vi "GetStatus.vi"(8 "error in (no error)":errorcluster, 11 "S4GUI in":refnum<class "S4GUI.lvclass">) -> (0 "error out":errorcluster, 3 "S4GUI out":refnum<class "S4GUI.lvclass">)   [LabVIEW 2018, in "S4GUI.lvclass"]
uses:
  S4GUI.lvclass
  S4GUI.lvclass/S4GUI.ctl
  Server/Server.lvclass/Server.ctl
  Instrument/Instrument.lvclass/Instrument.ctl
  Device/Optics/Optics.lvclass/Optics.ctl
  Interface/Interface.lvclass/Interface.ctl
  TelFocus/TelFocus.lvclass
  WeatherStation/WeatherStation.lvclass
  Instrument/Instrument.lvclass
  TCS/TCS.lvclass
  SyncBox/Sync Box.lvclass
  Device/Optics/Opt_Selector/Opt_Selector.lvclass
  Device/Optics/Opt_Continuous/Opt_Continuous.lvclass
  Acquisition/Acquisition.lvclass
  GSserver/GSserver.lvclass
  Channel/Channel.lvclass
  Interface/Interface.lvclass
  GSstatus/GSstatus.lvclass
  SecMirror/SecMirror.lvclass
  WeatherSensor/WeatherSensor.lvclass
  Trigger/Trigger.lvclass
  Device/Optics/Optics.lvclass
  Server/Server.lvclass
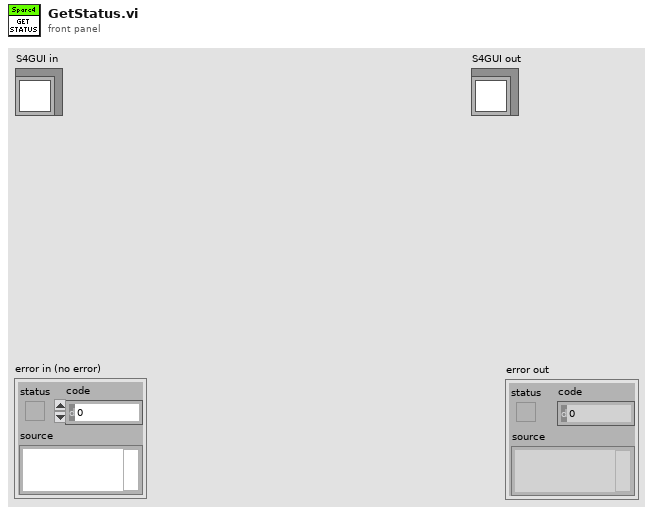
[diagram p1: front panel]
types:
  T1 = cluster{"ACQUISITION_MODE":bool, "TRIGGER_MODE":bool, "READ_MODE":bool, "PREAMP":bool, "READOUT_RATE":bool, "VERTICAL_SHIFT_SPEED":bool, "EM_MODE":bool, "EM_GAIN":bool, "SHUTTER_MODE":bool, "SHUTTER_TTL":bool, "SHUTTER_OPENING_TIME":bool, "SHUTTER_CLOSING_TIME":bool, "VBIN":bool, "HBIN":bool, "INITIAL_LINE":bool, "INITIAL_COLUMN":bool, "FINAL_LINE":bool, "FINAL_COLUMN":bool, "FRAME_TRANSFER":bool, "VERTICAL_CLOCK_VOLTAGE":bool, "AD_CHANNEL":bool}
  T2 = cluster{"ACQUISITION_MODE":u8, "TRIGGER_MODE":u8, "READ_MODE":u8, "PREAMP":u8, "READOUT_RATE":u8, "VERTICAL_SHIFT_SPEED":u8, "EM_MODE":u8, "EM_GAIN":u16, "SHUTTER_MODE":u8, "SHUTTER_TTL":u8, "SHUTTER_OPENING_TIME":u16, "SHUTTER_CLOSING_TIME":u16, "VBIN":u16, "HBIN":u16, "INITIAL_LINE":u16, "INITIAL_COLUMN":u16, "FINAL_LINE":u16, "FINAL_COLUMN":u16, "FRAME_TRANSFER":bool, "VERTICAL_CLOCK_VOLTAGE":u8, "AD_CHANNEL":u32}
  T3 = cluster{"Trigger Mode Status":string, "String output":string, "Instrument Status":cluster{"WPROT pos":dbl, "WPSEL pos":dbl, "GMIR pos":dbl, "GFOC pos":dbl, "CALW pos":dbl, "ASEL pos":dbl, "mode":bool, "String Status":string, "connection":bool, "operational":bool}, "Sync Box State":i32, "Trigger General Status":string, "Instrument States":cluster{"WPSEL State":i32, "WPROT State":i32, "CALW State":i32, "ASEL State":i32, "GMIR State":i32, "GFOC State":i32}, "Instrument Pos Names":cluster{"WPROT posname":string, "WPSEL posname":string, "CALW posname":string, "ASEL posname":string}, "ChannelA_Status":cluster{"Current exp":dbl, "Frames done":u32, "LastFileImage":string, "CamStatus":string, "Run state":u32, "connection":bool, "Cooler ON/OFF":i16, "Currently temperature":i16, "Temperature Status":string, "target  temp":i16, "conf runing":bool, "FT":bool, "UsedDisk":u16, "operational":bool}, "WPROT seq":u16, "ChannelB_Status":cluster{"Current exp":dbl, "Frames done":u32, "LastFileImage":string, "CamStatus":string, "Run state":u32, "connection":bool, "Cooler ON/OFF":i16, "Currently temperature":i16, "Temperature Status":string, "target  temp":i16, "conf runing":bool, "FT":bool, "UsedDisk":u16, "operational":bool}, "ChannelC_Status":cluster{"Current exp":dbl, "Frames done":u32, "LastFileImage":string, "CamStatus":string, "Run state":u32, "connection":bool, "Cooler ON/OFF":i16, "Currently temperature":i16, "Temperature Status":string, "target  temp":i16, "conf runing":bool, "FT":bool, "UsedDisk":u16, "operational":bool}, "ChannelD_Status":cluster{"Current exp":dbl, "Frames done":u32, "LastFileImage":string, "CamStatus":string, "Run state":u32, "connection":bool, "Cooler ON/OFF":i16, "Currently temperature":i16, "Temperature Status":string, "target  temp":i16, "conf runing":bool, "FT":bool, "UsedDisk":u16, "operational":bool}, "ChannelA_CCD":cluster{"ACQUISITION_MODE":u8, "TRIGGER_MODE":u8, "READ_MODE":u8, "PREAMP":u8, "READOUT_RATE":u8, "VERTICAL_SHIFT_SPEED":u8, "EM_MODE":u8, "EM_GAIN":u16, "SHUTTER_MODE":u8, "SHUTTER_TTL":u8, "SHUTTER_OPENNING_TIME":u16, "SHUTTER_CLOSING_TIME":u16, "VBIN":u16, "HBIN":u16, "INITIAL_LINE":u16, "INITIAL_COLUMN":u16, "FINAL_LINE":u16, "FINAL_COLUMN":u16, "FRAME_TRANSFER":bool, "VERTICAL_CLOCK_VOLTAGE":u8, "AD_CHANNEL":u32}, "ChannelB_CCD ":cluster{"ACQUISITION_MODE":u8, "TRIGGER_MODE":u8, "READ_MODE":u8, "PREAMP":u8, "READOUT_RATE":u8, "VERTICAL_SHIFT_SPEED":u8, "EM_MODE":u8, "EM_GAIN":u16, "SHUTTER_MODE":u8, "SHUTTER_TTL":u8, "SHUTTER_OPENNING_TIME":u16, "SHUTTER_CLOSING_TIME":u16, "VBIN":u16, "HBIN":u16, "INITIAL_LINE":u16, "INITIAL_COLUMN":u16, "FINAL_LINE":u16, "FINAL_COLUMN":u16, "FRAME_TRANSFER":bool, "VERTICAL_CLOCK_VOLTAGE":u8, "AD_CHANNEL":u32}, "ChannelC_CCD":cluster{"ACQUISITION_MODE":u8, "TRIGGER_MODE":u8, "READ_MODE":u8, "PREAMP":u8, "READOUT_RATE":u8, "VERTICAL_SHIFT_SPEED":u8, "EM_MODE":u8, "EM_GAIN":u16, "SHUTTER_MODE":u8, "SHUTTER_TTL":u8, "SHUTTER_OPENNING_TIME":u16, "SHUTTER_CLOSING_TIME":u16, "VBIN":u16, "HBIN":u16, "INITIAL_LINE":u16, "INITIAL_COLUMN":u16, "FINAL_LINE":u16, "FINAL_COLUMN":u16, "FRAME_TRANSFER":bool, "VERTICAL_CLOCK_VOLTAGE":u8, "AD_CHANNEL":u32}, "ChannelD_CCD":cluster{"ACQUISITION_MODE":u8, "TRIGGER_MODE":u8, "READ_MODE":u8, "PREAMP":u8, "READOUT_RATE":u8, "VERTICAL_SHIFT_SPEED":u8, "EM_MODE":u8, "EM_GAIN":u16, "SHUTTER_MODE":u8, "SHUTTER_TTL":u8, "SHUTTER_OPENNING_TIME":u16, "SHUTTER_CLOSING_TIME":u16, "VBIN":u16, "HBIN":u16, "INITIAL_LINE":u16, "INITIAL_COLUMN":u16, "FINAL_LINE":u16, "FINAL_COLUMN":u16, "FRAME_TRANSFER":bool, "VERTICAL_CLOCK_VOLTAGE":u8, "AD_CHANNEL":u32}, "CHA_Checked Params":cluster{"ACQUISITION_MODE":bool, "TRIGGER_MODE":bool, "READ_MODE":bool, "PREAMP":bool, "READOUT_RATE":bool, "VERTICAL_SHIFT_SPEED":bool, "EM_MODE":bool, "EM_GAIN":bool, "SHUTTER_MODE":bool, "SHUTTER_TTL":bool, "SHUTTER_OPENING_TIME":bool, "SHUTTER_CLOSING_TIME":bool, "VBIN":bool, "HBIN":bool, "INITIAL_LINE":bool, "INITIAL_COLUMN":bool, "FINAL_LINE":bool, "FINAL_COLUMN":bool, "FRAME_TRANSFER":bool, "VERTICAL_CLOCK_VOLTAGE":bool, "AD_CHANNEL":bool}, "CHB_Checked Params":cluster{"ACQUISITION_MODE":bool, "TRIGGER_MODE":bool, "READ_MODE":bool, "PREAMP":bool, "READOUT_RATE":bool, "VERTICAL_SHIFT_SPEED":bool, "EM_MODE":bool, "EM_GAIN":bool, "SHUTTER_MODE":bool, "SHUTTER_TTL":bool, "SHUTTER_OPENING_TIME":bool, "SHUTTER_CLOSING_TIME":bool, "VBIN":bool, "HBIN":bool, "INITIAL_LINE":bool, "INITIAL_COLUMN":bool, "FINAL_LINE":bool, "FINAL_COLUMN":bool, "FRAME_TRANSFER":bool, "VERTICAL_CLOCK_VOLTAGE":bool, "AD_CHANNEL":bool}, "CHC_Checked Params":cluster{"ACQUISITION_MODE":bool, "TRIGGER_MODE":bool, "READ_MODE":bool, "PREAMP":bool, "READOUT_RATE":bool, "VERTICAL_SHIFT_SPEED":bool, "EM_MODE":bool, "EM_GAIN":bool, "SHUTTER_MODE":bool, "SHUTTER_TTL":bool, "SHUTTER_OPENING_TIME":bool, "SHUTTER_CLOSING_TIME":bool, "VBIN":bool, "HBIN":bool, "INITIAL_LINE":bool, "INITIAL_COLUMN":bool, "FINAL_LINE":bool, "FINAL_COLUMN":bool, "FRAME_TRANSFER":bool, "VERTICAL_CLOCK_VOLTAGE":bool, "AD_CHANNEL":bool}, "CHD_Checked Params":cluster{"ACQUISITION_MODE":bool, "TRIGGER_MODE":bool, "READ_MODE":bool, "PREAMP":bool, "READOUT_RATE":bool, "VERTICAL_SHIFT_SPEED":bool, "EM_MODE":bool, "EM_GAIN":bool, "SHUTTER_MODE":bool, "SHUTTER_TTL":bool, "SHUTTER_OPENING_TIME":bool, "SHUTTER_CLOSING_TIME":bool, "VBIN":bool, "HBIN":bool, "INITIAL_LINE":bool, "INITIAL_COLUMN":bool, "FINAL_LINE":bool, "FINAL_COLUMN":bool, "FRAME_TRANSFER":bool, "VERTICAL_CLOCK_VOLTAGE":bool, "AD_CHANNEL":bool}, "Trigger_connection":bool, "TCSPD_connection":bool, "TCS extended":string, "TCS id":u32, "S4ICS id":u32, "focus pos":i32, "Focus_connection":bool, "WS_connection":bool, "weather status":cluster{"broker":string, "version":string, "date":string, "hour":string, "outHumidity":string, "inHumidity":string, "inTemp":string, "outTemp":string, "windSpeed":string, "windDirection":string, "pressure":string, "dewOut":string, "dewIn":string, "leaf":string, "rain":string, "windChill":string}, "GS STATUS cluster":cluster{"FocusPhot":dbl, "FocusPolar":dbl, "FocusEffic":dbl, "FocusInstrum":dbl, "ICS":bool, "AG":bool, "BROKER":string}, "TCSPD_operational":bool, "Focus_operational":bool, "object_suffix":string, "dflat_suffix":string, "sflat_suffix":string, "dark_suffix":string, "zero_suffix":string, "focus_suffix":string, "suffixAlertVisible":bool}
  T4 = cluster{"TEMP":dbl, "EXPTIME":dbl, "#FRAMES":u32, "#CYCLES":u32, "#SEQS":u32, "WAVEPLATE_POS":u32, "COOLER_POWER_STATUS":dbl, "suffix":string}
  T5 = cluster{"FocusPhot":dbl, "FocusPolar":dbl, "FocusEffic":dbl, "FocusInstrum":dbl, "ICS":bool, "AG":bool, "BROKER":string}
  T6 = cluster{"broker":string, "version":string, "date":string, "hour":string, "outHumidity":string, "intHumidity":string, "inTemp":string, "outTemp":string, "windSpeed":string, "windDirection":string, "pressure":string, "dewOut":string, "dewIn":string, "leaf":string, "rain":string, "windChill":string}
  T7 = cluster{"Texp":dbl, "Nimages":u32, "InitialLine":u32, "FinalLine":u32, "InitialColumn":u32, "FinalColumn":u32, "EmGain":u32, "Cooler Off":bool, "CyclesDone":u32, "SequesDone":u32, "UsedDiskSpace":u16, "Error":bool}
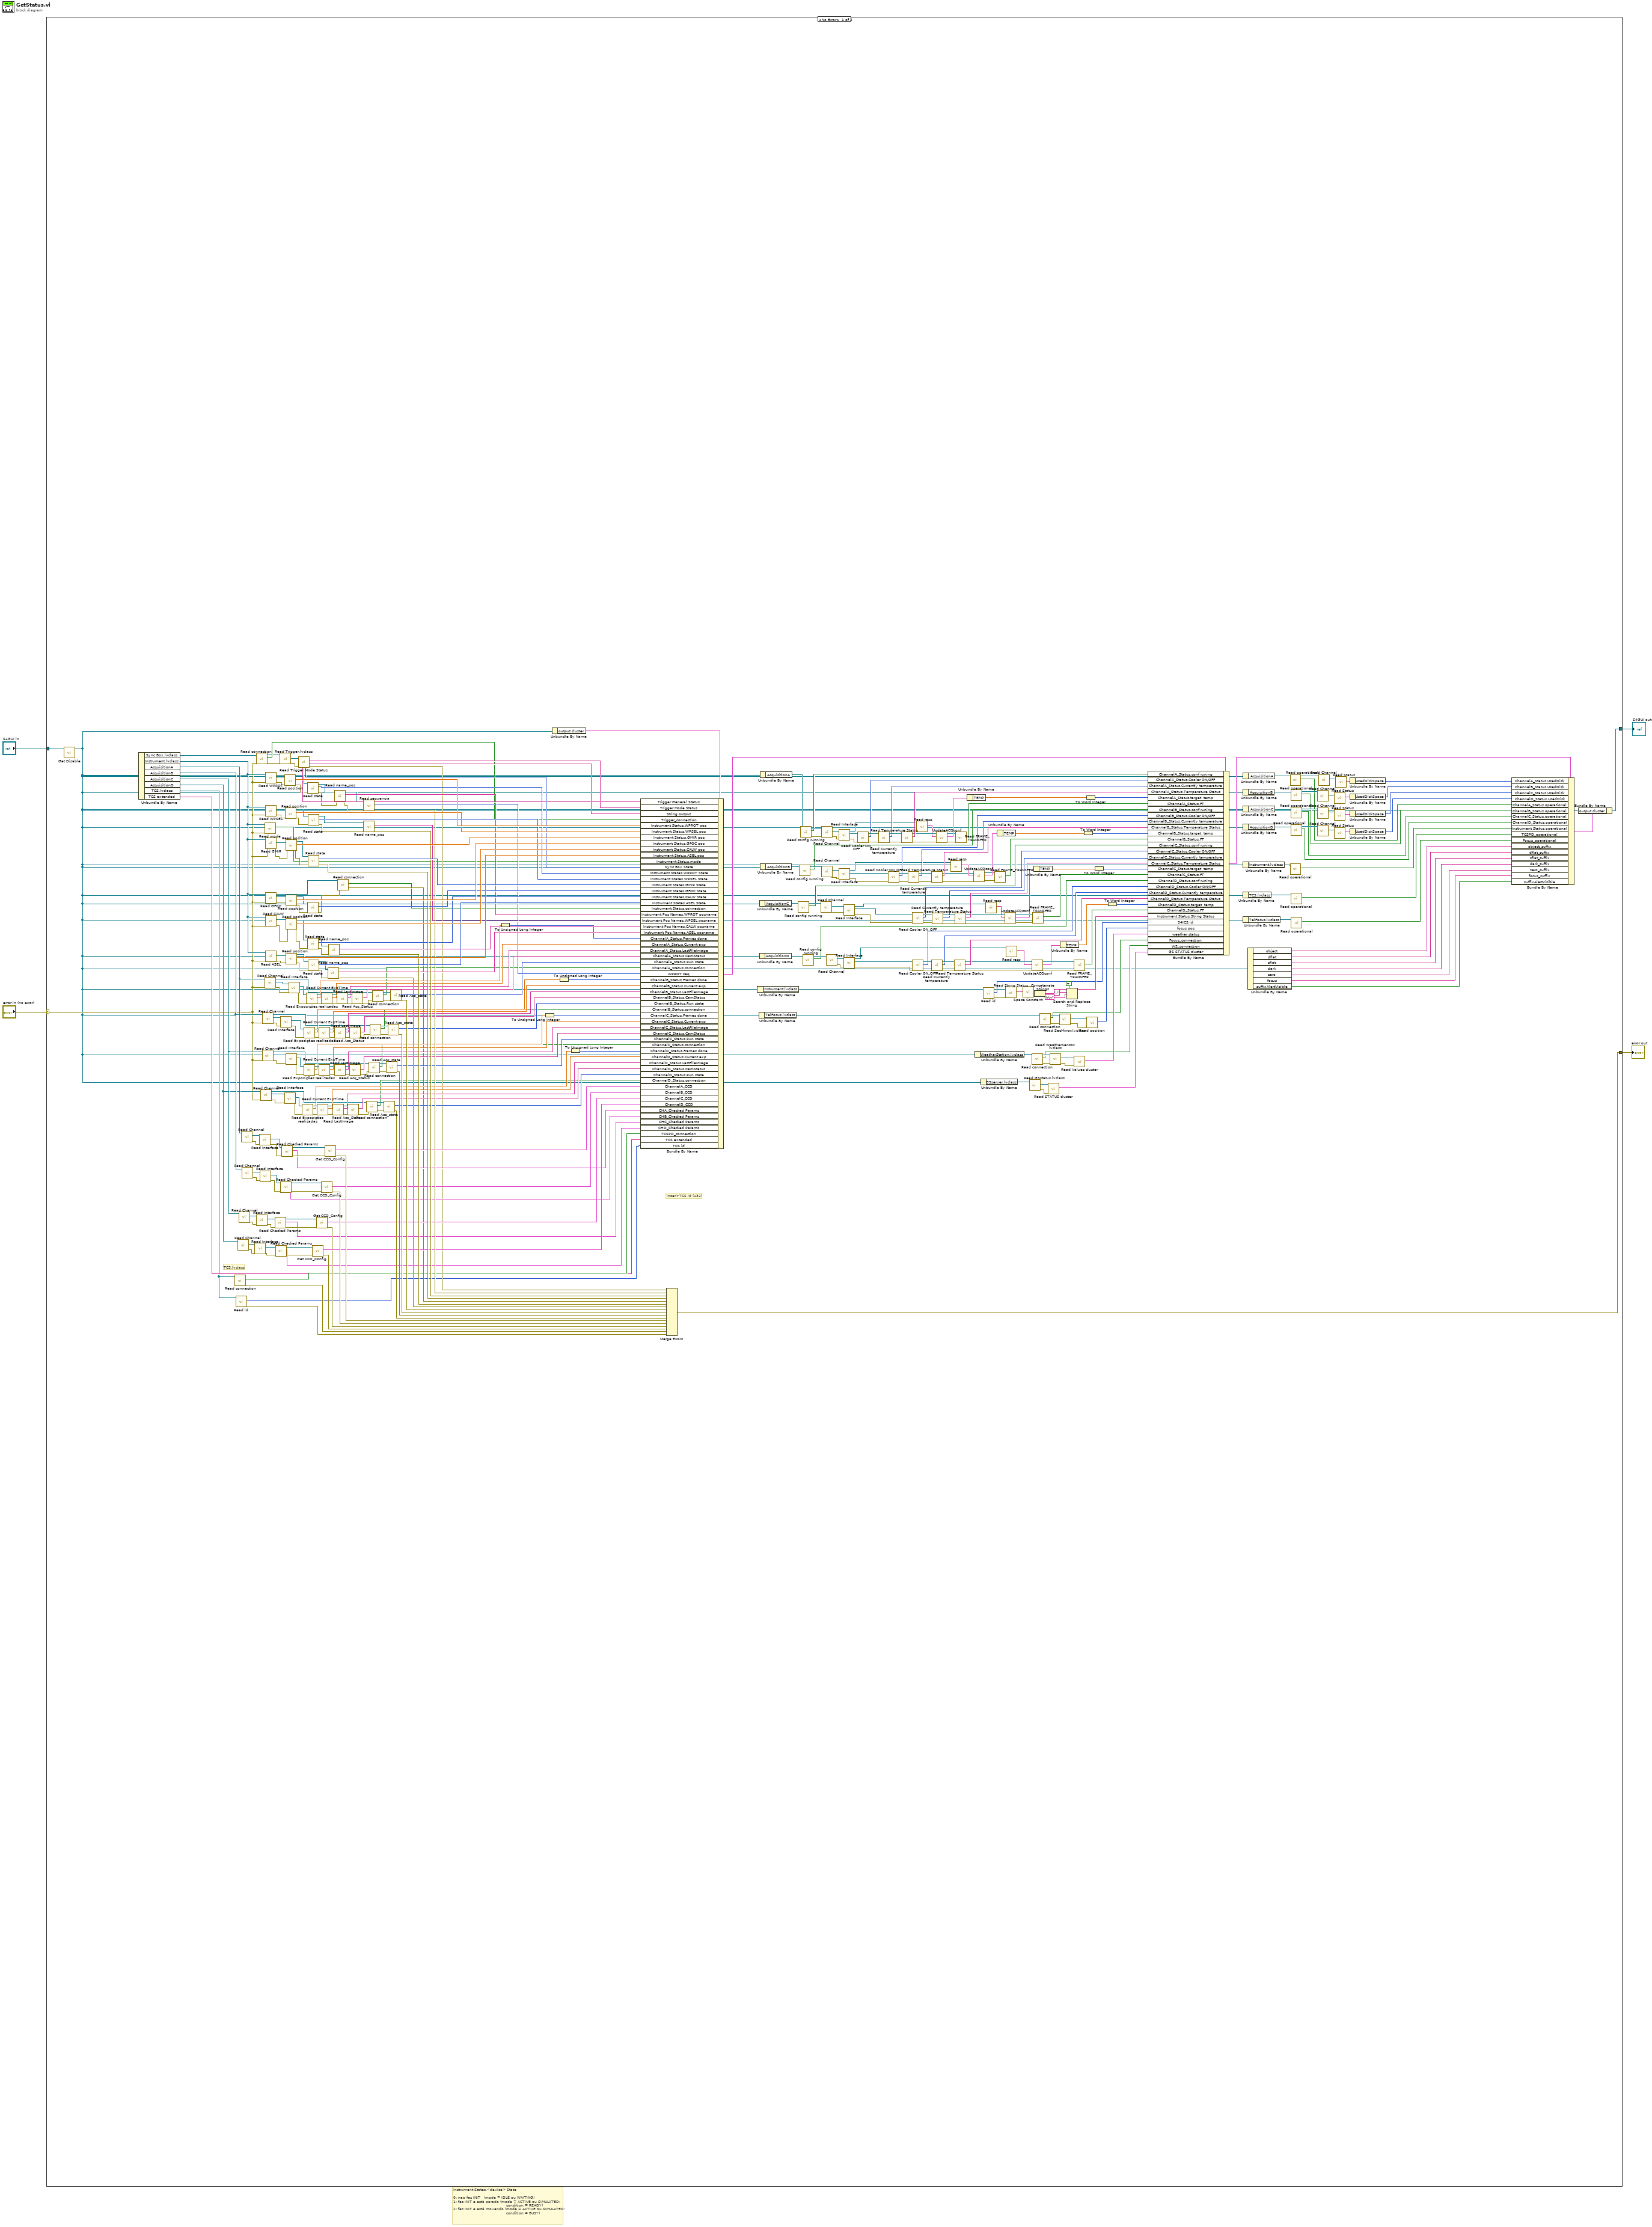
[diagram p0: block diagram]
diagram:
  # "Instrument States.<device> State\n\n0: nao fez INIT   (mode = IDLE ou WAITING)\n1: fez INIT e está parado (mode = ACTIVE ou SIMULATED;\n                                            condition = READY)\n2: fez INIT e está movendo (mode = ACTIVE ou SIMULATED;\n                                            condition = BUSY)"
  n1 = case shown="No Error" "error in (no error)" {
    selector: "error in (no error)" -> [w138 w385]
    tunnel: [w363 w385] -> w3
    tunnel: [w71 w384] -> w1
    tunnel: "S4GUI in" -> [w127 w384]
    frame No Error {
      # "inserir TCS id (U32)"
      # "TCS.lvclass"
      n2 = call-dynamic "Get Disable.vi"("S4ACS_GUI in"=w127) -> ("S4ACS_GUI out"=w12:refnum<class "S4GUI.lvclass">)  [unwired: 9 in, 1 out]
      n3 = Unbundle By Name(w12) -> ("Sync Box.lvclass"=w193:refnum<class "Sync Box.lvclass">, "Instrument.lvclass"=w139:refnum<class "Instrument.lvclass">, "AcquisitionA"=w252:refnum<class "Acquisition.lvclass">, "AcquisitionB"=w247:refnum<class "Acquisition.lvclass">, "AcquisitionC"=w242:refnum<class "Acquisition.lvclass">, "AcquisitionD"=w241:refnum<class "Acquisition.lvclass">, "TCS.lvclass"=w119:refnum<class "TCS.lvclass">, "TCS extended"=w120:string)
      n4 = call "Read connection.vi"("Server in"=w119) -> ("error out"=w117:errorcluster, "connection"=w184:bool)  [unwired: 8 in, 1 out]
      n5 = call "Read id.vi"("Server in"=w119) -> ("error out"=w118:errorcluster, "id"=w116:u32)  [unwired: 8 in, 1 out]
      n6 = call-dynamic "Read Channel.vi"("Acquisition in"=w241) -> ("error out"=w239:errorcluster, "Channel.lvclass"=w240:refnum<class "Channel.lvclass">)  [unwired: 8 in, 1 out]
      n7 = call-dynamic "Read Channel.vi"("Acquisition in"=w242) -> ("error out"=w244:errorcluster, "Channel.lvclass"=w243:refnum<class "Channel.lvclass">)  [unwired: 8 in, 1 out]
      n8 = call-dynamic "Read Channel.vi"("Acquisition in"=w252) -> ("error out"=w253:errorcluster, "Channel.lvclass"=w254:refnum<class "Channel.lvclass">)  [unwired: 8 in, 1 out]
      n9 = call-dynamic "Read Channel.vi"("Acquisition in"=w247) -> ("error out"=w249:errorcluster, "Channel.lvclass"=w248:refnum<class "Channel.lvclass">)  [unwired: 8 in, 1 out]
      n10 = call-dynamic "Read Interface.vi"("error in (no error)"=w239, "Channel in"=w240) -> ("error out"=w221:errorcluster, "Interface.lvclass"=w222:refnum<class "Interface.lvclass">)  [unwired: 7 in, 1 out]
      n11 = call-dynamic "Read Interface.vi"("error in (no error)"=w244, "Channel in"=w243) -> ("error out"=w225:errorcluster, "Interface.lvclass"=w223:refnum<class "Interface.lvclass">)  [unwired: 7 in, 1 out]
      n12 = call "Read connection.vi"("error in (no error)"=w138, "Server in"=w193) -> ("error out"=w190:errorcluster, "connection"=w194:bool, "Server out"=w192:refnum<class "Sync Box.lvclass">)  [unwired: 7 in]
      n13 = call-dynamic "Read Interface.vi"("error in (no error)"=w253, "Channel in"=w254) -> ("error out"=w234:errorcluster, "Interface.lvclass"=w232:refnum<class "Interface.lvclass">)  [unwired: 7 in, 1 out]
      n14 = call-dynamic "Read Interface.vi"("error in (no error)"=w249, "Channel in"=w248) -> ("error out"=w229:errorcluster, "Interface.lvclass"=w227:refnum<class "Interface.lvclass">)  [unwired: 7 in, 1 out]
      n15 = call-dynamic "Read Channel.vi"("error in (no error)"=w138, "Acquisition in"=w241) -> ("error out"=w270:errorcluster, "Channel.lvclass"=w269:refnum<class "Channel.lvclass">, "Acquisition out"=w198:refnum<class "Acquisition.lvclass">)  [unwired: 7 in]
      n16 = call-dynamic "Read Channel.vi"("error in (no error)"=w138, "Acquisition in"=w242) -> ("error out"=w280:errorcluster, "Channel.lvclass"=w279:refnum<class "Channel.lvclass">, "Acquisition out"=w202:refnum<class "Acquisition.lvclass">)  [unwired: 7 in]
      n17 = call-dynamic "Read Channel.vi"("error in (no error)"=w138, "Acquisition in"=w247) -> ("error out"=w297:errorcluster, "Channel.lvclass"=w296:refnum<class "Channel.lvclass">, "Acquisition out"=w206:refnum<class "Acquisition.lvclass">)  [unwired: 7 in]
      n18 = call-dynamic "Read mode.vi"("error in (no error)"=w138, "Instrument in"=w139) -> ("mode"=w137:bool)  [unwired: 7 in, 2 out]
      n19 = call-dynamic "Read Channel.vi"("error in (no error)"=w138, "Acquisition in"=w252) -> ("error out"=w325:errorcluster, "Channel.lvclass"=w326:refnum<class "Channel.lvclass">, "Acquisition out"=w214:refnum<class "Acquisition.lvclass">)  [unwired: 7 in]
      n20 = call "Read WPROT.vi"("error in (no error)"=w138, "Instrument in"=w139) -> ("error out"=w379:errorcluster, "Opt_Selector.lvclass"=w380:refnum<class "Opt_Selector.lvclass">)  [unwired: 7 in, 1 out]
      n21 = call "Read WPSEL.vi"("error in (no error)"=w138, "Instrument in"=w139) -> ("error out"=w381:errorcluster, "Opt_Selector.lvclass"=w378:refnum<class "Opt_Selector.lvclass">)  [unwired: 7 in, 1 out]
      n22 = call "Read GMIR.vi"("error in (no error)"=w138, "Instrument in"=w139) -> ("error out"=w377:errorcluster, "Opt_Continuous.lvclass"=w375:refnum<class "Opt_Continuous.lvclass">)  [unwired: 7 in, 1 out]
      n23 = call "Read GFOC.vi"("error in (no error)"=w138, "Instrument in"=w139) -> ("error out"=w373:errorcluster, "Opt_Continuous.lvclass"=w374:refnum<class "Opt_Continuous.lvclass">, "Instrument out"=w217:refnum<class "Instrument.lvclass">)  [unwired: 7 in]
      n24 = call "Read CALW.vi"("error in (no error)"=w138, "Instrument in"=w139) -> ("error out"=w376:errorcluster, "Opt_Selector.lvclass"=w372:refnum<class "Opt_Selector.lvclass">)  [unwired: 7 in, 1 out]
      n25 = call "Read ASEL.vi"("error in (no error)"=w138, "Instrument in"=w139) -> ("error out"=w371:errorcluster, "Opt_Selector.lvclass"=w370:refnum<class "Opt_Selector.lvclass">)  [unwired: 7 in, 1 out]
      n26 = call "Read Checked Params.vi"("error in (no error)"=w225, "Interface in"=w223) -> ("error out"=w224:errorcluster, "Checked Params"=w208:T1, "Interface out"=w218:refnum<class "Interface.lvclass">)  [unwired: 7 in]
      n27 = call "Read Checked Params.vi"("error in (no error)"=w221, "Interface in"=w222) -> ("error out"=w220:errorcluster, "Checked Params"=w207:T1, "Interface out"=w219:refnum<class "Interface.lvclass">)  [unwired: 7 in]
      n28 = call-dynamic "Read Trigger.lvclass.vi"("error in (no error)"=w190, "Sync Box in"=w192) -> ("error out"=w189:errorcluster, "Trigger.lvclass"=w191:refnum<class "Trigger.lvclass">)  [unwired: 7 in, 1 out]
      n29 = call-dynamic "Read Interface.vi"("error in (no error)"=w297, "Channel in"=w296) -> ("error out"=w302:errorcluster, "Interface.lvclass"=w298:refnum<class "Interface.lvclass">)  [unwired: 7 in, 1 out]
      n30 = call "Read Checked Params.vi"("error in (no error)"=w229, "Interface in"=w227) -> ("error out"=w228:errorcluster, "Checked Params"=w209:T1, "Interface out"=w226:refnum<class "Interface.lvclass">)  [unwired: 7 in]
      n31 = call "Read Checked Params.vi"("error in (no error)"=w234, "Interface in"=w232) -> ("error out"=w233:errorcluster, "Checked Params"=w230:T1, "Interface out"=w231:refnum<class "Interface.lvclass">)  [unwired: 7 in]
      n32 = call-dynamic "Read Interface.vi"("error in (no error)"=w270, "Channel in"=w269) -> ("error out"=w275:errorcluster, "Interface.lvclass"=w271:refnum<class "Interface.lvclass">)  [unwired: 7 in, 1 out]
      n33 = call "Read position.vi"("error in (no error)"=w379, "Optics in"=w380) -> ("error out"=w359:errorcluster, "position"=w369:dbl, "Optics out"=w360:refnum<class "Opt_Selector.lvclass">)  [unwired: 7 in]
      n34 = call "Read position.vi"("error in (no error)"=w381, "Optics in"=w378) -> ("error out"=w356:errorcluster, "position"=w368:dbl, "Optics out"=w357:refnum<class "Opt_Selector.lvclass">)  [unwired: 7 in]
      n35 = call "Read position.vi"("error in (no error)"=w377, "Optics in"=w375) -> ("error out"=w353:errorcluster, "position"=w367:dbl, "Optics out"=w354:refnum<class "Opt_Continuous.lvclass">)  [unwired: 7 in]
      n36 = call "Read position.vi"("error in (no error)"=w373, "Optics in"=w374) -> ("error out"=w349:errorcluster, "position"=w366:dbl, "Optics out"=w350:refnum<class "Opt_Continuous.lvclass">)  [unwired: 7 in]
      n37 = call "Read position.vi"("error in (no error)"=w371, "Optics in"=w370) -> ("error out"=w343:errorcluster, "position"=w364:dbl, "Optics out"=w344:refnum<class "Opt_Selector.lvclass">)  [unwired: 7 in]
      n38 = call "Read position.vi"("error in (no error)"=w376, "Optics in"=w372) -> ("error out"=w346:errorcluster, "position"=w365:dbl, "Optics out"=w347:refnum<class "Opt_Selector.lvclass">)  [unwired: 7 in]
      n39 = call-dynamic "Read Interface.vi"("error in (no error)"=w280, "Channel in"=w279) -> ("error out"=w285:errorcluster, "Interface.lvclass"=w281:refnum<class "Interface.lvclass">)  [unwired: 7 in, 1 out]
      n40 = call-dynamic "Read Interface.vi"("error in (no error)"=w325, "Channel in"=w326) -> ("error out"=w315:errorcluster, "Interface.lvclass"=w324:refnum<class "Interface.lvclass">)  [unwired: 7 in, 1 out]
      n41 = call-dynamic "Read Trigger Mode Status.vi"("error in (no error)"=w189, "Trigger in"=w191) -> ("error out"=w188:errorcluster, "String output"=w382:string, "Trigger Mode Status"=w383:string, "State"=w362:i32, "Trigger General Status"=w361:string)  [unwired: 4 in, 1 out]
      n42 = call-dynamic "Read Exposições realizadas.vi"("error in (no error)"=w275, "Interface in"=w271) -> ("error out"=w276:errorcluster, "Exposições realizadas"=w261:dbl, "Interface out"=w272:refnum<class "Interface.lvclass">)  [unwired: 7 in]
      n43 = call-dynamic "Read Exposições realizadas.vi"("error in (no error)"=w285, "Interface in"=w281) -> ("error out"=w286:errorcluster, "Exposições realizadas"=w268:dbl, "Interface out"=w282:refnum<class "Interface.lvclass">)  [unwired: 7 in]
      n44 = call-dynamic "Read Exposições realizadas.vi"("error in (no error)"=w302, "Interface in"=w298) -> ("error out"=w303:errorcluster, "Exposições realizadas"=w294:dbl, "Interface out"=w299:refnum<class "Interface.lvclass">)  [unwired: 7 in]
      n45 = call-dynamic "Read Exposições realizadas.vi"("error in (no error)"=w315, "Interface in"=w324) -> ("error out"=w314:errorcluster, "Exposições realizadas"=w319:dbl, "Interface out"=w323:refnum<class "Interface.lvclass">)  [unwired: 7 in]
      n46 = call-dynamic "Read state.vi"("error in (no error)"=w359, "Optics in"=w360) -> ("error out"=w341:errorcluster, "state"=w358:u8, "Optics out"=w340:refnum<class "Opt_Selector.lvclass">)  [unwired: 7 in]
      n47 = call-dynamic "Read state.vi"("error in (no error)"=w349, "Optics in"=w350) -> ("error out"=w216:errorcluster, "state"=w348:u8)  [unwired: 7 in, 1 out]
      n48 = call-dynamic "Read state.vi"("error in (no error)"=w346, "Optics in"=w347) -> ("error out"=w334:errorcluster, "state"=w345:u8, "Optics out"=w332:refnum<class "Opt_Selector.lvclass">)  [unwired: 7 in]
      n49 = call-dynamic "Read state.vi"("error in (no error)"=w356, "Optics in"=w357) -> ("error out"=w337:errorcluster, "state"=w355:u8, "Optics out"=w336:refnum<class "Opt_Selector.lvclass">)  [unwired: 7 in]
      n50 = call-dynamic "Read state.vi"("error in (no error)"=w353, "Optics in"=w354) -> ("error out"=w352:errorcluster, "state"=w351:u8)  [unwired: 7 in, 1 out]
      n51 = call-dynamic "Read state.vi"("error in (no error)"=w343, "Optics in"=w344) -> ("error out"=w330:errorcluster, "state"=w342:u8, "Optics out"=w328:refnum<class "Opt_Selector.lvclass">)  [unwired: 7 in]
      n52 = call-dynamic "Get CCD_Config.vi"("error in (no error)"=w220, "Interface in"=w219) -> ("error out"=w235:errorcluster, "output cluster"=w237:T2)  [unwired: 7 in, 1 out]
      n53 = call-dynamic "Get CCD_Config.vi"("error in (no error)"=w224, "Interface in"=w218) -> ("error out"=w236:errorcluster, "output cluster"=w238:T2)  [unwired: 7 in, 1 out]
      n54 = call-dynamic "Read Current ExpTime.vi"("error in (no error)"=w276, "Interface in"=w272) -> ("error out"=w277:errorcluster, "Current ExpTime"=w259:dbl, "Interface out"=w273:refnum<class "Interface.lvclass">)  [unwired: 7 in]
      n55 = call-dynamic "Read Current ExpTime.vi"("error in (no error)"=w286, "Interface in"=w282) -> ("error out"=w287:errorcluster, "Current ExpTime"=w266:dbl, "Interface out"=w283:refnum<class "Interface.lvclass">)  [unwired: 7 in]
      n56 = call-dynamic "Read Current ExpTime.vi"("error in (no error)"=w303, "Interface in"=w299) -> ("error out"=w304:errorcluster, "Current ExpTime"=w292:dbl, "Interface out"=w300:refnum<class "Interface.lvclass">)  [unwired: 7 in]
      n57 = call-dynamic "Read Current ExpTime.vi"("error in (no error)"=w314, "Interface in"=w323) -> ("error out"=w313:errorcluster, "Current ExpTime"=w320:dbl, "Interface out"=w322:refnum<class "Interface.lvclass">)  [unwired: 7 in]
      n58 = call-dynamic "Get CCD_Config.vi"("error in (no error)"=w228, "Interface in"=w226) -> ("error out"=w246:errorcluster, "output cluster"=w245:T2)  [unwired: 7 in, 1 out]
      n59 = call-dynamic "Get CCD_Config.vi"("error in (no error)"=w233, "Interface in"=w231) -> ("error out"=w250:errorcluster, "output cluster"=w251:T2)  [unwired: 7 in, 1 out]
      n60 = call "Read name_pos.vi"("error in (no error)"=w330, "Optics in"=w328) -> ("error out"=w329:errorcluster, "name_pos"=w327:string)  [unwired: 7 in, 1 out]
      n61 = call "Read name_pos.vi"("error in (no error)"=w334, "Optics in"=w332) -> ("error out"=w333:errorcluster, "name_pos"=w331:string)  [unwired: 7 in, 1 out]
      n62 = call-dynamic "Read LastImage.vi"("error in (no error)"=w277, "Interface in"=w273) -> ("error out"=w278:errorcluster, "LastImage"=w258:string, "Interface out"=w274:refnum<class "Interface.lvclass">)  [unwired: 7 in]
      n63 = call-dynamic "Read LastImage.vi"("error in (no error)"=w287, "Interface in"=w283) -> ("error out"=w288:errorcluster, "LastImage"=w265:string, "Interface out"=w284:refnum<class "Interface.lvclass">)  [unwired: 7 in]
      n64 = call "Read name_pos.vi"("error in (no error)"=w341, "Optics in"=w340) -> ("error out"=w310:errorcluster, "name_pos"=w339:string, "Optics out"=w311:refnum<class "Opt_Selector.lvclass">)  [unwired: 7 in]
      n65 = call-dynamic "Read LastImage.vi"("error in (no error)"=w304, "Interface in"=w300) -> ("error out"=w305:errorcluster, "LastImage"=w291:string, "Interface out"=w301:refnum<class "Interface.lvclass">)  [unwired: 7 in]
      n66 = call-dynamic "Read LastImage.vi"("error in (no error)"=w313, "Interface in"=w322) -> ("error out"=w312:errorcluster, "LastImage"=w317:string, "Interface out"=w321:refnum<class "Interface.lvclass">)  [unwired: 7 in]
      n67 = call "Read connection.vi"("error in (no error)"=w216, "Server in"=w217) -> ("error out"=w215:errorcluster, "connection"=w68:bool)  [unwired: 7 in, 1 out]
      n68 = call-dynamic "Read Acq_Status.vi"("error in (no error)"=w278, "Interface in"=w274) -> ("error out"=w197:errorcluster, "Acq_Status"=w257:string)  [unwired: 7 in, 1 out]
      n69 = call-dynamic "Read Acq_Status.vi"("error in (no error)"=w288, "Interface in"=w284) -> ("error out"=w200:errorcluster, "Acq_Status"=w264:string)  [unwired: 7 in, 1 out]
      n70 = call-dynamic "Read Acq_Status.vi"("error in (no error)"=w305, "Interface in"=w301) -> ("error out"=w204:errorcluster, "Acq_Status"=w290:string)  [unwired: 7 in, 1 out]
      n71 = call-dynamic "Read Acq_Status.vi"("error in (no error)"=w312, "Interface in"=w321) -> ("error out"=w212:errorcluster, "Acq_Status"=w316:string)  [unwired: 7 in, 1 out]
      n72 = call-dynamic "Read sequencia.vi"("error in (no error)"=w310, "Opt_Selector in"=w311) -> ("error out"=w309:errorcluster, "sequencia"=w308:u16)  [unwired: 7 in, 1 out]
      n73 = call "Read name_pos.vi"("error in (no error)"=w337, "Optics in"=w336) -> ("error out"=w338:errorcluster, "name_pos"=w335:string)  [unwired: 7 in, 1 out]
      n74 = call "Read connection.vi"("error in (no error)"=w197, "Server in"=w198) -> ("error out"=w196:errorcluster, "connection"=w185:bool, "Server out"=w195:refnum<class "Acquisition.lvclass">)  [unwired: 7 in]
      n75 = call "Read connection.vi"("error in (no error)"=w200, "Server in"=w202) -> ("error out"=w199:errorcluster, "connection"=w186:bool, "Server out"=w201:refnum<class "Acquisition.lvclass">)  [unwired: 7 in]
      n76 = call "Read connection.vi"("error in (no error)"=w204, "Server in"=w206) -> ("error out"=w203:errorcluster, "connection"=w187:bool, "Server out"=w205:refnum<class "Acquisition.lvclass">)  [unwired: 7 in]
      n77 = call "Read connection.vi"("error in (no error)"=w212, "Server in"=w214) -> ("error out"=w211:errorcluster, "connection"=w210:bool, "Server out"=w213:refnum<class "Acquisition.lvclass">)  [unwired: 7 in]
      n78 = call-dynamic "Read Acq_state.vi"("error in (no error)"=w196, "Acquisition in"=w195) -> ("error out"=w255:errorcluster, "Acq_state"=w256:u32)  [unwired: 7 in, 1 out]
      n79 = call-dynamic "Read Acq_state.vi"("error in (no error)"=w199, "Acquisition in"=w201) -> ("error out"=w262:errorcluster, "Acq_state"=w263:u32)  [unwired: 7 in, 1 out]
      n80 = call-dynamic "Read Acq_state.vi"("error in (no error)"=w203, "Acquisition in"=w205) -> ("error out"=w295:errorcluster, "Acq_state"=w289:u32)  [unwired: 7 in, 1 out]
      n81 = call-dynamic "Read Acq_state.vi"("error in (no error)"=w211, "Acquisition in"=w213) -> ("error out"=w306:errorcluster, "Acq_state"=w307:u32)  [unwired: 7 in, 1 out]
      n82 = To Unsigned Long Integer(number=w319) -> (unsigned 32bit integer=w318:u32)
      n83 = To Unsigned Long Integer(number=w268) -> (unsigned 32bit integer=w267:u32)
      n84 = Unbundle By Name(w12) -> ("output cluster"=w70:T3)
      n85 = To Unsigned Long Integer(number=w294) -> (unsigned 32bit integer=w293:u32)
      n86 = To Unsigned Long Integer(number=w261) -> (unsigned 32bit integer=w260:u32)
      n87 = Bundle By Name(cluster=w70, "Trigger General Status"=w361, "Trigger Mode Status"=w383, "String output"=w382, "Trigger_connection"=w194, "Instrument Status.WPROT pos"=w369, "Instrument Status.WPSEL pos"=w368, "Instrument Status.GMIR pos"=w367, "Instrument Status.GFOC pos"=w366, "Instrument Status.CALW pos"=w365, "Instrument Status.ASEL pos"=w364, "Instrument Status.mode"=w137, "Sync Box State"=w362, "Instrument States.WPROT State"=w358, "Instrument States.WPSEL State"=w355, "Instrument States.GMIR State"=w351, "Instrument States.GFOC State"=w348, "Instrument States.CALW State"=w345, "Instrument States.ASEL State"=w342, "Instrument Status.connection"=w68, "Instrument Pos Names.WPROT posname"=w339, "Instrument Pos Names.WPSEL posname"=w335, "Instrument Pos Names.CALW posname"=w331, "Instrument Pos Names.ASEL posname"=w327, "ChannelA_Status.Frames done"=w318, "ChannelA_Status.Current exp"=w320, "ChannelA_Status.LastFileImage"=w317, "ChannelA_Status.CamStatus"=w316, "ChannelA_Status.Run state"=w307, "ChannelA_Status.connection"=w210, "WPROT seq"=w308, "ChannelB_Status.Frames done"=w293, "ChannelB_Status.Current exp"=w292, "ChannelB_Status.LastFileImage"=w291, "ChannelB_Status.CamStatus"=w290, "ChannelB_Status.Run state"=w289, "ChannelB_Status.connection"=w187, "ChannelC_Status.Frames done"=w267, "ChannelC_Status.Current exp"=w266, "ChannelC_Status.LastFileImage"=w265, "ChannelC_Status.CamStatus"=w264, "ChannelC_Status.Run state"=w263, "ChannelC_Status.connection"=w186, "ChannelD_Status.Frames done"=w260, "ChannelD_Status.Current exp"=w259, "ChannelD_Status.LastFileImage"=w258, "ChannelD_Status.CamStatus"=w257, "ChannelD_Status.Run state"=w256, "ChannelD_Status.connection"=w185, "ChannelA_CCD"=w251, "ChannelB_CCD"=w245, "ChannelC_CCD"=w238, "ChannelD_CCD"=w237, "CHA_Checked Params"=w230, "CHB_Checked Params"=w209, "CHC_Checked Params"=w208, "CHD_Checked Params"=w207, "TCSPD_connection"=w184, "TCS extended"=w120, "TCS id"=w116) -> (w69:T3)
      n88 = Merge Errors(w188, w309, w338, w352, w215, w333, w329, w306, w295, w262, w255, w250, w246, w236, w235, w117, w118) -> (w363:errorcluster)
      n89 = Unbundle By Name(w12) -> ("Instrument.lvclass"=w106:refnum<class "Instrument.lvclass">)
      n90 = Unbundle By Name(w12) -> ("TelFocus.lvclass"=w96:refnum<class "TelFocus.lvclass">)
      n91 = Unbundle By Name(w12) -> ("AcquisitionC"=w124:refnum<class "Acquisition.lvclass">)
      n92 = Unbundle By Name(w12) -> ("AcquisitionD"=w122:refnum<class "Acquisition.lvclass">)
      n93 = Unbundle By Name(w12) -> ("AcquisitionA"=w129:refnum<class "Acquisition.lvclass">)
      n94 = Unbundle By Name(w12) -> ("AcquisitionB"=w126:refnum<class "Acquisition.lvclass">)
      n95 = call-dynamic "Read config running.vi"("Server in"=w124) -> ("config running"=w110:bool, "Server out"=w123:refnum<class "Acquisition.lvclass">)  [unwired: 8 in, 1 out]
      n96 = call-dynamic "Read config running.vi"("Server in"=w126) -> ("config running"=w111:bool, "Server out"=w125:refnum<class "Acquisition.lvclass">)  [unwired: 8 in, 1 out]
      n97 = call-dynamic "Read config running.vi"("Server in"=w129) -> ("error out"=w112:errorcluster, "config running"=w113:bool, "Server out"=w128:refnum<class "Acquisition.lvclass">)  [unwired: 8 in]
      n98 = call-dynamic "Read config running.vi"("Server in"=w122) -> ("config running"=w108:bool, "Server out"=w121:refnum<class "Acquisition.lvclass">)  [unwired: 8 in, 1 out]
      n99 = call-dynamic "Read Channel.vi"("Acquisition in"=w123) -> ("error out"=w176:errorcluster, "Channel.lvclass"=w177:refnum<class "Channel.lvclass">)  [unwired: 8 in, 1 out]
      n100 = call-dynamic "Read Channel.vi"("error in (no error)"=w112, "Acquisition in"=w128) -> ("error out"=w182:errorcluster, "Channel.lvclass"=w183:refnum<class "Channel.lvclass">)  [unwired: 7 in, 1 out]
      n101 = call-dynamic "Read Channel.vi"("Acquisition in"=w125) -> ("error out"=w179:errorcluster, "Channel.lvclass"=w180:refnum<class "Channel.lvclass">)  [unwired: 8 in, 1 out]
      n102 = call-dynamic "Read Channel.vi"("Acquisition in"=w121) -> ("error out"=w173:errorcluster, "Channel.lvclass"=w174:refnum<class "Channel.lvclass">)  [unwired: 8 in, 1 out]
      n103 = call-dynamic "Read Interface.vi"("error in (no error)"=w182, "Channel in"=w183) -> ("error out"=w166:errorcluster, "Interface.lvclass"=w181:refnum<class "Interface.lvclass">, "Channel out"=w43:refnum<class "Channel.lvclass">)  [unwired: 7 in]
      n104 = call-dynamic "Read Interface.vi"("error in (no error)"=w179, "Channel in"=w180) -> ("error out"=w160:errorcluster, "Interface.lvclass"=w178:refnum<class "Interface.lvclass">, "Channel out"=w39:refnum<class "Channel.lvclass">)  [unwired: 7 in]
      n105 = call-dynamic "Read Interface.vi"("error in (no error)"=w176, "Channel in"=w177) -> ("error out"=w150:errorcluster, "Interface.lvclass"=w175:refnum<class "Interface.lvclass">, "Channel out"=w25:refnum<class "Channel.lvclass">)  [unwired: 7 in]
      n106 = call-dynamic "Read Interface.vi"("error in (no error)"=w173, "Channel in"=w174) -> ("error out"=w149:errorcluster, "Interface.lvclass"=w172:refnum<class "Interface.lvclass">, "Channel out"=w17:refnum<class "Channel.lvclass">)  [unwired: 7 in]
      n107 = call-dynamic "Read Cooler ON_OFF.vi"("error in (no error)"=w166, "Interface in"=w181) -> ("error out"=w165:errorcluster, "Cooler ON/OFF"=w169:i16, "Interface out"=w171:refnum<class "Interface.lvclass">)  [unwired: 7 in]
      n108 = call-dynamic "Read Currently temperature.vi"("error in (no error)"=w165, "Interface in"=w171) -> ("error out"=w164:errorcluster, "Currently temperature"=w168:i8, "Interface out"=w170:refnum<class "Interface.lvclass">)  [unwired: 7 in]
      n109 = call-dynamic "Read Cooler ON_OFF.vi"("error in (no error)"=w160, "Interface in"=w178) -> ("error out"=w161:errorcluster, "Cooler ON/OFF"=w158:i16, "Interface out"=w159:refnum<class "Interface.lvclass">)  [unwired: 7 in]
      n110 = call-dynamic "Read Temperature Status.vi"("error in (no error)"=w164, "Interface in"=w170) -> ("error out"=w46:errorcluster, "Temperature Status"=w167:string, "Interface out"=w47:refnum<class "Interface.lvclass">)  [unwired: 7 in]
      n111 = call-dynamic "Read Currently temperature.vi"("error in (no error)"=w161, "Interface in"=w159) -> ("error out"=w162:errorcluster, "Currently temperature"=w157:i8, "Interface out"=w163:refnum<class "Interface.lvclass">)  [unwired: 7 in]
      n112 = call-dynamic "Read Cooler ON_OFF.vi"("error in (no error)"=w150, "Interface in"=w175) -> ("error out"=w151:errorcluster, "Cooler ON/OFF"=w145:i16, "Interface out"=w153:refnum<class "Interface.lvclass">)  [unwired: 7 in]
      n113 = call-dynamic "Read Cooler ON_OFF.vi"("error in (no error)"=w149, "Interface in"=w172) -> ("error out"=w148:errorcluster, "Cooler ON/OFF"=w142:i16, "Interface out"=w147:refnum<class "Interface.lvclass">)  [unwired: 7 in]
      n114 = call-dynamic "Read resp.vi"("Device in"=w43) -> ("resp"=w42:string)  [unwired: 8 in, 2 out]
      n115 = call-dynamic "Read Temperature Status.vi"("error in (no error)"=w162, "Interface in"=w163) -> ("error out"=w34:errorcluster, "Temperature Status"=w156:string, "Interface out"=w35:refnum<class "Interface.lvclass">)  [unwired: 7 in]
      n116 = call-dynamic "Read Currently temperature.vi"("error in (no error)"=w148, "Interface in"=w147) -> ("error out"=w154:errorcluster, "Currently temperature"=w141:i8, "Interface out"=w146:refnum<class "Interface.lvclass">)  [unwired: 7 in]
      n117 = call-dynamic "Read Currently temperature.vi"("error in (no error)"=w151, "Interface in"=w153) -> ("error out"=w155:errorcluster, "Currently temperature"=w144:i8, "Interface out"=w152:refnum<class "Interface.lvclass">)  [unwired: 7 in]
      n118 = call-dynamic "UpdateACQconf.vi"("error in (no error)"=w46, "status"=w42, "Interface in"=w47) -> ("error out"=w40:errorcluster, "ACQ conf rx"=w48:T4, "Interface out"=w41:refnum<class "Interface.lvclass">)  [unwired: 6 in]
      n119 = call-dynamic "Read resp.vi"("Device in"=w39) -> ("resp"=w38:string)  [unwired: 8 in, 2 out]
      n120 = call-dynamic "Read Temperature Status.vi"("error in (no error)"=w154, "Interface in"=w146) -> ("error out"=w20:errorcluster, "Temperature Status"=w140:string, "Interface out"=w21:refnum<class "Interface.lvclass">)  [unwired: 7 in]
      n121 = call-dynamic "Read Temperature Status.vi"("error in (no error)"=w155, "Interface in"=w152) -> ("error out"=w27:errorcluster, "Temperature Status"=w143:string, "Interface out"=w29:refnum<class "Interface.lvclass">)  [unwired: 7 in]
      n122 = call-dynamic "Read FRAME_TRANSFER.vi"("error in (no error)"=w40, "Interface in"=w41) -> ("FRAME_TRANSFER"=w115:bool)  [unwired: 7 in, 2 out]
      n123 = Unbundle By Name(w48) -> ("TEMP"=w45:dbl)
      n124 = call-dynamic "UpdateACQconf.vi"("error in (no error)"=w34, "status"=w38, "Interface in"=w35) -> ("error out"=w31:errorcluster, "ACQ conf rx"=w37:T4, "Interface out"=w32:refnum<class "Interface.lvclass">)  [unwired: 6 in]
      n125 = Unbundle By Name(w12) -> ("WeatherStation.lvclass"=w92:refnum<class "WeatherStation.lvclass">)
      n126 = Unbundle By Name(w12) -> ("GSserver.lvclass"=w88:refnum<class "GSserver.lvclass">)
      n127 = call "Read id.vi"("Server in"=w106) -> ("error out"=w103:errorcluster, "id"=w104:u32, "Server out"=w105:refnum<class "Instrument.lvclass">)  [unwired: 8 in]
      n128 = call-dynamic "Read resp.vi"("Device in"=w25) -> ("resp"=w24:string)  [unwired: 8 in, 2 out]
      n129 = call-dynamic "Read FRAME_TRANSFER.vi"("error in (no error)"=w31, "Interface in"=w32) -> ("FRAME_TRANSFER"=w114:bool)  [unwired: 7 in, 2 out]
      n130 = Unbundle By Name(w37) -> ("TEMP"=w36:dbl)
      n131 = call-dynamic "UpdateACQconf.vi"("error in (no error)"=w27, "status"=w24, "Interface in"=w29) -> ("error out"=w26:errorcluster, "ACQ conf rx"=w23:T4, "Interface out"=w28:refnum<class "Interface.lvclass">)  [unwired: 6 in]
      n132 = call-dynamic "Read String Status.vi"("error in (no error)"=w103, "Server in"=w105) -> ("String Status"=w132:string)  [unwired: 7 in, 2 out]
      n133 = call-dynamic "Read resp.vi"("Device in"=w17) -> ("resp"=w16:string)  [unwired: 8 in, 2 out]
      n134 = call <vilib>:"Space Constant.vi"() -> ("String"=w133:string)
      n135 = call-dynamic "Read GSstatus.lvclass.vi"("GSserver in"=w88) -> ("error out"=w86:errorcluster, "GSstatus.lvclass"=w87:refnum<class "GSstatus.lvclass">)  [unwired: 8 in, 1 out]
      n136 = call "Read connection.vi"("Server in"=w92) -> ("error out"=w90:errorcluster, "connection"=w89:bool, "Server out"=w91:refnum<class "WeatherStation.lvclass">)  [unwired: 8 in]
      n137 = call-dynamic "UpdateACQconf.vi"("error in (no error)"=w20, "status"=w16, "Interface in"=w21) -> ("error out"=w18:errorcluster, "ACQ conf rx"=w15:T4, "Interface out"=w19:refnum<class "Interface.lvclass">)  [unwired: 6 in]
      n138 = call-dynamic "Read FRAME_TRANSFER.vi"("error in (no error)"=w26, "Interface in"=w28) -> ("FRAME_TRANSFER"=w109:bool)  [unwired: 7 in, 2 out]
      n139 = Unbundle By Name(w23) -> ("TEMP"=w30:dbl)
      n140 = Concatenate Strings(w133, w132) -> (w131:string)
      n141 = call "Read connection.vi"("Server in"=w96) -> ("error out"=w94:errorcluster, "connection"=w93:bool, "Server out"=w95:refnum<class "TelFocus.lvclass">)  [unwired: 8 in]
      n142 = call-dynamic "Read STATUS cluster.vi"("error in (no error)"=w86, "GSstatus in"=w87) -> ("STATUS cluster"=w85:T5)  [unwired: 7 in, 2 out]
      n143 = call-dynamic "Read WeatherSensor.lvclass.vi"("error in (no error)"=w90, "WeatherStation in"=w91) -> ("error out"=w99:errorcluster, "WeatherSensor.lvclass"=w100:refnum<class "WeatherSensor.lvclass">)  [unwired: 7 in, 1 out]
      n144 = call-dynamic "Read SecMirror.lvclass.vi"("error in (no error)"=w94, "TelFocus in"=w95) -> ("error out"=w101:errorcluster, "SecMirror.lvclass"=w102:refnum<class "SecMirror.lvclass">)  [unwired: 7 in, 1 out]
      n145 = Unbundle By Name(w15) -> ("TEMP"=w14:dbl)
      n146 = Search and Replace String(replace all?=TRUE ("replace all? (F)"), input string=w131, search string=",", replace string="\r\n" ("input string")) -> (result string=w130:string)  [unwired: 4 in, 3 out]
      n147 = call-dynamic "Read FRAME_TRANSFER.vi"("error in (no error)"=w18, "Interface in"=w19) -> ("FRAME_TRANSFER"=w107:bool)  [unwired: 7 in, 2 out]
      n148 = call-dynamic "Read Values cluster.vi"("error in (no error)"=w99, "WeatherSensor in"=w100) -> ("Values cluster"=w97:T6)  [unwired: 7 in, 2 out]
      n149 = To Word Integer(number=w36) -> (16bit integer=w33:i16)
      n150 = To Word Integer(number=w45) -> (16bit integer=w44:i16)
      n151 = call-dynamic "Read position.vi"("error in (no error)"=w101, "SecMirror in"=w102) -> ("position"=w98:i32)  [unwired: 7 in, 2 out]
      n152 = To Word Integer(number=w30) -> (16bit integer=w22:i16)
      n153 = To Word Integer(number=w14) -> (16bit integer=w13:i16)
      n154 = Bundle By Name(cluster=w69, "ChannelA_Status.conf runing"=w113, "ChannelA_Status.Cooler ON/OFF"=w169, "ChannelA_Status.Currently temperature"=w168, "ChannelA_Status.Temperature Status"=w167, "ChannelA_Status.target  temp"=w44, "ChannelA_Status.FT"=w115, "ChannelB_Status.conf runing"=w111, "ChannelB_Status.Cooler ON/OFF"=w158, "ChannelB_Status.Currently temperature"=w157, "ChannelB_Status.Temperature Status"=w156, "ChannelB_Status.target  temp"=w33, "ChannelB_Status.FT"=w114, "ChannelC_Status.conf runing"=w110, "ChannelC_Status.Cooler ON/OFF"=w145, "ChannelC_Status.Currently temperature"=w144, "ChannelC_Status.Temperature Status"=w143, "ChannelC_Status.target  temp"=w22, "ChannelC_Status.FT"=w109, "ChannelD_Status.conf runing"=w108, "ChannelD_Status.Cooler ON/OFF"=w142, "ChannelD_Status.Currently temperature"=w141, "ChannelD_Status.Temperature Status"=w140, "ChannelD_Status.target  temp"=w13, "ChannelD_Status.FT"=w107, "Instrument Status.String Status"=w130, "S4ICS id"=w104, "focus pos"=w98, "weather status"=w97, "Focus_connection"=w93, "WS_connection"=w89, "GS STATUS cluster"=w85) -> (w75:T3)
      n155 = Unbundle By Name(w12) -> ("AcquisitionA"=w67:refnum<class "Acquisition.lvclass">)
      n156 = Unbundle By Name(w12) -> ("AcquisitionB"=w65:refnum<class "Acquisition.lvclass">)
      n157 = Unbundle By Name(w12) -> ("AcquisitionC"=w63:refnum<class "Acquisition.lvclass">)
      n158 = Unbundle By Name(w12) -> ("AcquisitionD"=w61:refnum<class "Acquisition.lvclass">)
      n159 = Unbundle By Name(w12) -> ("Instrument.lvclass"=w59:refnum<class "Instrument.lvclass">)
      n160 = Unbundle By Name(w12) -> ("TCS.lvclass"=w58:refnum<class "TCS.lvclass">)
      n161 = Unbundle By Name(w12) -> ("TelFocus.lvclass"=w57:refnum<class "TelFocus.lvclass">)
      n162 = Unbundle By Name(w12) -> ("object"=w11:string, "dflat"=w10:string, "sflat"=w9:string, "dark"=w8:string, "zero"=w7:string, "focus"=w6:string, "suffixAlertVisible"=w5:bool)
      n163 = call-dynamic "Read operational.vi"("Server in"=w67) -> ("operational"=w56:bool, "Server out"=w66:refnum<class "Acquisition.lvclass">)  [unwired: 8 in, 1 out]
      n164 = call-dynamic "Read operational.vi"("Server in"=w59) -> ("operational"=w52:bool)  [unwired: 8 in, 2 out]
      n165 = call-dynamic "Read operational.vi"("Server in"=w65) -> ("operational"=w55:bool, "Server out"=w64:refnum<class "Acquisition.lvclass">)  [unwired: 8 in, 1 out]
      n166 = call-dynamic "Read operational.vi"("Server in"=w63) -> ("operational"=w54:bool, "Server out"=w62:refnum<class "Acquisition.lvclass">)  [unwired: 8 in, 1 out]
      n167 = call-dynamic "Read operational.vi"("Server in"=w61) -> ("operational"=w53:bool, "Server out"=w60:refnum<class "Acquisition.lvclass">)  [unwired: 8 in, 1 out]
      n168 = call-dynamic "Read operational.vi"("Server in"=w58) -> ("operational"=w51:bool)  [unwired: 8 in, 2 out]
      n169 = call-dynamic "Read operational.vi"("Server in"=w57) -> ("operational"=w50:bool)  [unwired: 8 in, 2 out]
      n170 = call-dynamic "Read Channel.vi"("Acquisition in"=w64) -> ("Channel.lvclass"=w81:refnum<class "Channel.lvclass">)  [unwired: 8 in, 2 out]
      n171 = call-dynamic "Read Channel.vi"("Acquisition in"=w62) -> ("Channel.lvclass"=w79:refnum<class "Channel.lvclass">)  [unwired: 8 in, 2 out]
      n172 = call-dynamic "Read Channel.vi"("Acquisition in"=w60) -> ("Channel.lvclass"=w77:refnum<class "Channel.lvclass">)  [unwired: 8 in, 2 out]
      n173 = call-dynamic "Read Channel.vi"("Acquisition in"=w66) -> ("Channel.lvclass"=w84:refnum<class "Channel.lvclass">)  [unwired: 8 in, 2 out]
      n174 = call-dynamic "Read Status.vi"("Channel in"=w81) -> ("Status"=w80:T7)  [unwired: 8 in, 2 out]
      n175 = call-dynamic "Read Status.vi"("Channel in"=w79) -> ("Status"=w78:T7)  [unwired: 8 in, 2 out]
      n176 = call-dynamic "Read Status.vi"("Channel in"=w77) -> ("Status"=w76:T7)  [unwired: 8 in, 2 out]
      n177 = call-dynamic "Read Status.vi"("Channel in"=w84) -> ("Status"=w83:T7)  [unwired: 8 in, 2 out]
      n178 = Unbundle By Name(w83) -> ("UsedDiskSpace"=w82:u16)
      n179 = Unbundle By Name(w80) -> ("UsedDiskSpace"=w74:u16)
      n180 = Unbundle By Name(w78) -> ("UsedDiskSpace"=w73:u16)
      n181 = Unbundle By Name(w76) -> ("UsedDiskSpace"=w72:u16)
      n182 = Bundle By Name(cluster=w75, "ChannelA_Status.UsedDisk"=w82, "ChannelB_Status.UsedDisk"=w74, "ChannelC_Status.UsedDisk"=w73, "ChannelD_Status.UsedDisk"=w72, "ChannelA_Status.operational"=w56, "ChannelB_Status.operational"=w55, "ChannelC_Status.operational"=w54, "ChannelD_Status.operational"=w53, "Instrument Status.operational"=w52, "TCSPD_operational"=w51, "Focus_operational"=w50, "object_suffix"=w11, "dflat_suffix"=w10, "sflat_suffix"=w9, "dark_suffix"=w8, "zero_suffix"=w7, "focus_suffix"=w6, "suffixAlertVisible"=w5) -> (w49:T3)
      n183 = Bundle By Name(cluster=w12, "output cluster"=w49) -> (w71:refnum<class "S4GUI.lvclass">)
    }
    frame Error {
    }
  }
  "error out" <- w3
  "S4GUI out" <- w1
